vi "ISX3_Cmd_GetChannel.vi"() -> (0 "get Setup Channel config":u8[](array[numeric]))   [LabVIEW 2012, in "Sciospec ISX3 Impedance Analyzer.lvlib"]
uses:
  Sciospec ISX3 Impedance Analyzer.lvlib
panel:
  # "This VI generates the command to read\nthe channel and the range setting"
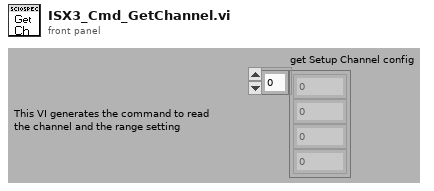
[diagram p1: front panel]
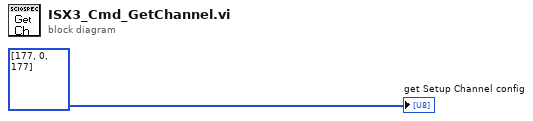
[diagram p0: block diagram]
diagram:
  "get Setup Channel config" <- u8[] [177, 0, 177]
